vi "setUp.vi"(8 "error in (no error)":errorcluster, 11 "reference in":refnum<class "Common System Tests.lvclass">) -> (0 "error out":errorcluster, 3 "reference out":refnum<class "Common System Tests.lvclass">)   [LabVIEW 2019, in "Common System Tests.lvclass"]
doc: "setUp runs prior to the test method during test execution. Use this method to initialize any object data required by your tests."
uses:
  Common System Tests.lvclass
  C:/Program Files (x86)/National Instruments/LabVIEW 2019/vi.lib/addons/_JKI Toolkits/VI Tester/TestCase.llb/TestCase.lvclass
  Assets/TCP_Listener.vi
  <vilib>/addons/_JKI Toolkits/VI Tester/TestCase.llb/TestCase.lvclass
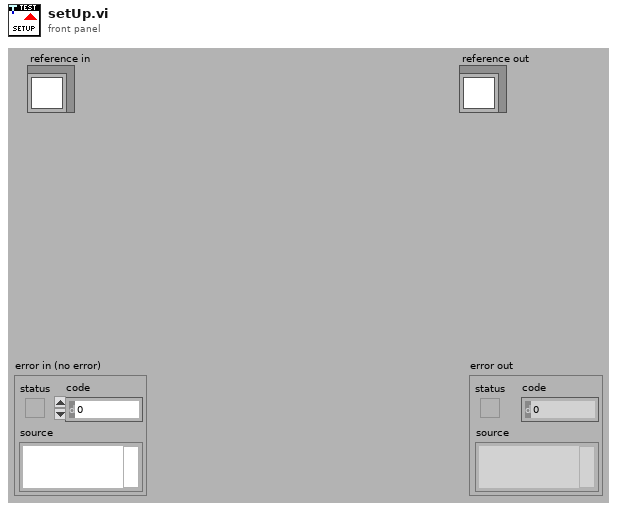
[diagram p1: front panel]
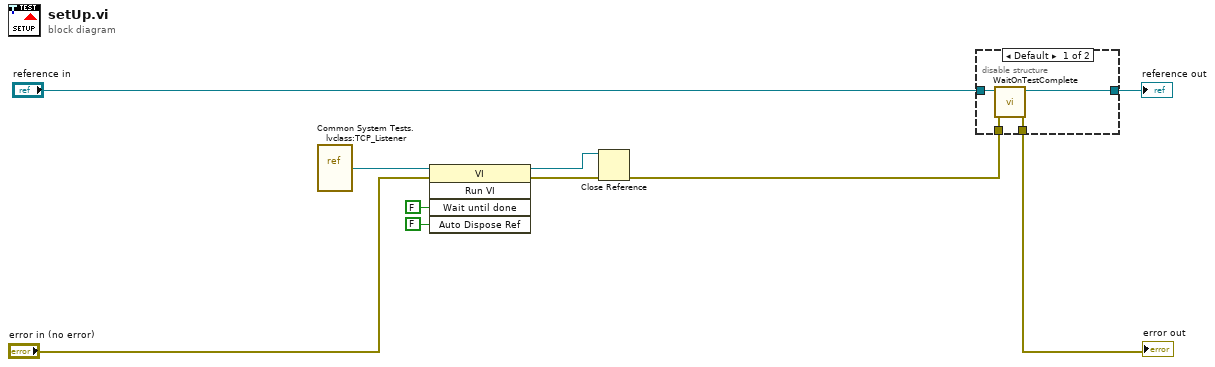
[diagram p0: block diagram]
diagram:
  n1 = vi-ref "Common System Tests.lvclass:TCP_Listener.vi"() -> (w7:refnum<vi>)
  n2 = invoke class="VI" method="Run VI"(reference=w7, error in="error in (no error)", "Wait until done"=FALSE ("Wait Until Done"), "Auto Dispose Ref"=FALSE ("Auto Dispose Reference")) -> (reference out=w5:refnum<vi>, error out=w4:errorcluster)  [unwired: 1 in, 3 out]
  n3 = Close Reference(reference=w5, error in (no error)=w4) -> (error out=w3:errorcluster)
  n4 = disable-structure shown="Default" {
    disable-tunnel: w3 -> [w14 w15]
    disable-tunnel: [w13 w15] -> w10
    disable-tunnel: [w12 w16] -> w9
    disable-tunnel: "reference in" -> [w11 w16]
    frame condition #0 (active) {
      n5 = call <vilib>:"WaitOnTestComplete.vi"("error in (no error)"=w14, "TestCase in"=w11) -> ("error out"=w13:errorcluster, "TestCase out"=w12:refnum<class "Common System Tests.lvclass">)  [unwired: 8 in]
    }
    frame condition #1 {
    }
  }
  "error out" <- w10
  "reference out" <- w9
